vi "Raman Live Tool Set v10.0.0.vi"(1 "Exit":bool, 2 "LiveData":dbl[][](array[numeric]), 3 "RemoteIndicator":bool) -> ()   [LabVIEW 2010]
uses:
  subvi/_TypeDefs/MapFunctions.ctl
  <vilib>/Utility/miscctls.llb/LVPointTypeDef.ctl
  <vilib>/Utility/miscctls.llb/LVStringsAndValuesArrayTypeDef.ctl
  <vilib>/Utility/inputDevices.llb/closeKeyboard.vi
  <vilib>/Utility/inputDevices.llb/keyboardAcquire.vi
  <vilib>/Utility/file.llb/Read From Spreadsheet File (DBL).vi
  <vilib>/Analysis/NI_AALBase.lvlib
panel:
  out "XY Full Interpol.":cluster{dbl, dbl}[](array[cluster])
  out "Axes":T1
  in  "SpectrumNoise":dbl caption="Noise?"
  in  "MapFunction":T2 caption="Mapping function" items=["Total"=0, "Peak"=4, "Area"=2, "Value"=1, "Ratio"=3]
  in  "CreateMap":bool
  in  "SpectrumX":u16(ring) caption="X"
  in  "SpectrumY":u16(ring) caption="Y"
  out "Spectrum":cluster{dbl[], dbl[]}(graph) caption="Current Spectrum"
  in  "MapKeyboard":bool
  in  "MapEditColor":bool caption="Edit Color"
  in  "MapFlipColor":bool caption="Flip Color"
  in  "MapInterpolate":bool
  in  "MapSaveData":bool
  out "Map":dbl[][](graph)
  out "LoadingSpectra":bool
  in  "SourceFile":path caption="Mapping File"
  in  "MapCursorDummy":bool
  out "XY Unique":cluster{"X Unique":dbl[], "Y Unique":dbl[]}
  out "XY Full":cluster{dbl, dbl}[](array[cluster])
  out "Intensities (2D)":dbl[][](array[numeric])
  out "Wavelengths (1D)":dbl[](array[numeric])
  in  "MapColorSlider":cluster{i32, i32, i32, i32, i32, i32, i32}(slide) scale=-6.0..134.0
  out "MapColorTable":u32[](array[numeric])=[0, 196608, 393216, 589824, 786432, 983040, 1179648, 1376256, 1572864, 1769472, 1966080, 2162688, 2359296, 2555904, 2752512, 2949120, 3145728, 3342336, 3538944, 3735552, 3932160, 4128768, 4325376, 4521984, 4718592, 4915200, 5111808, 5308416, 5505024, 5701632, 5898240, 6094848, 6291456, 6488064, 6684672, 6881280, 7077888, 7274496, 7471104, 7667712, 7864320, 8060928, 8257536, 8454144, 8650752, 8847360, 9043968, 9240576, 9437184, 9633792, 9830400, 10027008, 10223616, 10420224, 10616832, 10813440, 11010048, 11206656, 11403264, 11599872, 11796480, 11993088, 12189696, 12386304, 12582912, 12779520, 12976128, 13172736, 13369344, 13565952, 13762560, 13959168, 14155776, 14352384, 14548992, 14745600, 14942208, 15138816, 15335424, 15532032, 15728640, 15925248, 16121856, 16318464, 16515072, 16711680, 16712448, 16713216, 16713984, 16714752, 16715520, 16716288, 16717056, 16717824, 16718592, 16719360, 16720128, 16720896, 16721664, 16722432, 16723200, 16723968, 16724736, 16725504, 16726272, 16727040, 16727808, 16728576, 16729344, 16730112, 16730880, 16731648, 16732416, 16733184, 16733952, 16734720, 16735488, 16736256, 16737024, 16737792, 16738560, 16739328, 16740096, 16740864, 16741632, 16742400, 16743168, 16743936, 16744704, 16745472, 16746240, 16747008, 16747776, 16748544, 16749312, 16750080, 16750848, 16751616, 16752384, 16753152, 16753920, 16754688, 16755456, 16756224, 16756992, 16757760, 16758528, 16759296, 16760064, 16760832, 16761600, 16762368, 16763136, 16763904, 16764672, 16765440, 16766208, 16766976, 16767744, 16768512, 16769280, 16770048, 16770816, 16771584, 16772352, 16773120, 16773888, 16774656, 16775424, 16776192, 16776960, 16776963, 16776966, 16776969, 16776972, 16776975, 16776977, 16776980, 16776983, 16776986, 16776989, 16776992, 16776995, 16776998, 16777001, 16777004, 16777007, 16777009, 16777012, 16777015, 16777018, 16777021, 16777024, 16777027, 16777030, 16777033, 16777036, 16777038, 16777041, 16777044, 16777047, 16777050, 16777053, 16777056, 16777059, 16777062, 16777065, 16777068, 16777070, 16777073, 16777076, 16777079, 16777082, 16777085, 16777088, 16777091, 16777094, 16777097, 16777100, 16777102, 16777105, 16777108, 16777111, 16777114, 16777117, 16777120, 16777123, 16777126, 16777129, 16777132, 16777134, 16777137, 16777140, 16777143, 16777146, 16777149, 16777152, 16777155, 16777158, 16777161, 16777163, 16777166, 16777169, 16777172, 16777175, 16777178, 16777181, 16777184, 16777187, 16777190, 16777193, 16777195, 16777198, 16777201, 16777204, 16777207]
  out "MapZBounds":cluster{dbl, dbl}
  out "MapData (2D)":dbl[][](array[numeric])
  # "Cursor"
  # "Spectrum"
  # "Raman Live Tool Set"
  # "by A. Schmitz-Wunderlich, P. Candeloro"
  # "Cursor"
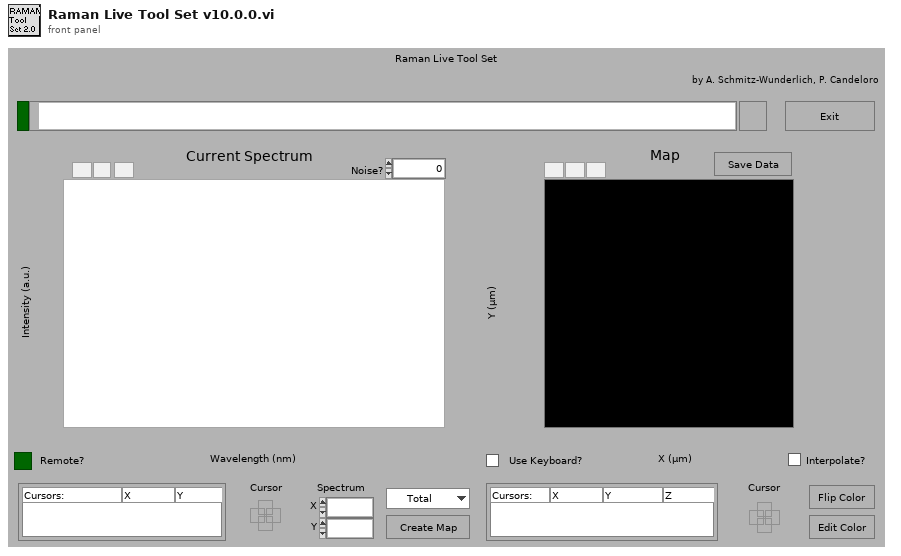
[diagram p1: front panel]
types:
  T1 = cluster{"X":cluster{"Offset":dbl, "Step Size":dbl, "Step Count":i32}, "Y":cluster{"Offset":dbl, "Step Size":dbl, "Step Count":i32}}
  T2 = typedef "MapFunctions.ctl" = u16
  T3 = typedef "LVPointTypeDef.ctl" = cluster{"Horizontal":i16, "Vertical":i16}
  T4 = enum8{"Enabled", "Disabled", "Disabled and Grayed Out"}
  T5 = enum16{"0", "1", "2", "3", "4", "5", "6", "7", "8", "9", "A", "B", "C", "D", "E", "F", "G", "H", "I", "J", "K", "L", "M", "N", "O", "P", "Q", "R", "S", "T", "U", "V", "W", "X", "Y", "Z", "F1", "F2", "F3", "F4", "F5", "F6", "F7", "F8", "F9", "F10", "F11", "F12", "F13", "F14", "F15", "ADD", "BACK", "BACKSLASH", "CAPITAL", "COMMA", "DECIMAL", "DELETE", "DIVIDE", "DOWN", "END", "EQUALS", "ESCAPE", "GRAVE (`)", "HOME", "INSERT", "LBRACKET", "LCONTROL", "LEFT", "L ALT", "LSHIFT", "LWIN", "MINUS", "MULTIPLY", "NEXT", "NUMLOCK", "NUMPAD_0", "NUMPAD_1", "NUMPAD_2", "NUMPAD_3", "NUMPAD_4", "NUMPAD_5", "NUMPAD_6", "NUMPAD_7", "NUMPAD_8", "NUMPAD_9", "PAUSE", "PERIOD", "PRIOR (PG UP)", "RBRACKET", "RCONTROL", "RETURN", "RIGHT", "R ALT", "RSHIFT", "RWIN", "SCROLL", "SEMICOLON", "SLASH", "SPACE", "SUBTRACT", "TAB", "UP", "ENTER (num pad)", "' (quote)"}
  T6 = enum16{"0", "1", "2", "3", "4", "5", "6", "7", "8", "9", "A", "B", "C", "D", "E", "F", "G", "H", "I", "J", "K", "L", "M", "N", "O", "P", "Q", "R", "S", "T", "U", "V", "W", "X", "Y", "Z", "F1", "F2", "F3", "F4", "F5", "F6", "F7", "F8", "F9", "F10", "F11", "F12", "F13", "F14", "F15", "ADD", "BACK", "BACKSLASH", "CAPITAL", "COMMA", "DECIMAL", "DELETE", "DIVIDE", "DOWN", "END", "EQUALS", "ESCAPE", "GRAVE (`)", "HOME", "INSERT", "LBRACKET", "LCONTROL", "LEFT", "L ALT", "LSHIFT", "LWIN", "MINUS", "MULTIPLY", "NEXT", "NUMLOCK", "NUMPAD_0", "NUMPAD_1", "NUMPAD_2", "NUMPAD_3", "NUMPAD_4", "NUMPAD_5", "NUMPAD_6", "NUMPAD_7", "NUMPAD_8", "NUMPAD_9", "PAUSE", "PERIOD", "PRIOR (PG UP)", "RBRACKET", "RCONTROL", "RETURN", "RIGHT", "R ALT", "RSHIFT", "RWIN", "SCROLL", "SEMICOLON", "SLASH", "SPACE", "SUBTRACT", "TAB", "UP", "ENTER (num pad)", "' (quote)"}[]
  T7 = cluster{"Name":string, "Color":u32, "Style":u8, "Point Style":u8, "Name Visible":bool, "Allow Drag":bool, "Cursor Mode":u32, "Plot":i32, "Index":i32, "Position":cluster{"X":dbl, "Y":dbl}, "X Scale":u32, "Y Scale":u32, "Watch Plots":i32[], "Watch All Plots":bool, "Plot Area":i32, "Label Offset":cluster{"X":dbl, "Y":dbl}}
  T8 = cluster{"Name":string, "Color":u32, "Style":u8, "Point Style":u8, "Name Visible":bool, "Allow Drag":bool, "Cursor Mode":u32, "Plot":i32, "Index":i32, "Position":cluster{"X":dbl, "Y":dbl}, "X Scale":u32, "Y Scale":u32, "Watch Plots":i32[], "Watch All Plots":bool, "Plot Area":i32, "Label Offset":cluster{"X":dbl, "Y":dbl}}[]
  T9 = typedef "LVCursorListTypeDef.ctl" = cluster{"Name":string, "Color":u32, "Style":u8, "Point Style":u8, "Name Visible":bool, "Allow Drag":bool, "Cursor Mode":u32, "Plot":i32, "Index":i32, "Position":cluster{"X":dbl, "Y":dbl}, "X Scale":u32, "Y Scale":u32, "Watch Plots":i32[], "Watch All Plots":bool, "Plot Area":i32, "Label Offset":cluster{"X":dbl, "Y":dbl}}[]
  T10 = typedef "LVPointDoubleTypeDef.ctl" = cluster{"Cursor X":dbl, "Cursor Y":dbl}
  T11 = typedef "LVStringsAndValuesArrayTypeDef.ctl" = cluster{"String":string, "Value":ext}[]
  T12 = enum32{"invalid app kind", "Development System", "Run Time System", "Student Edition", "Embedded LabVIEW", "Evaluation", "Custom"}
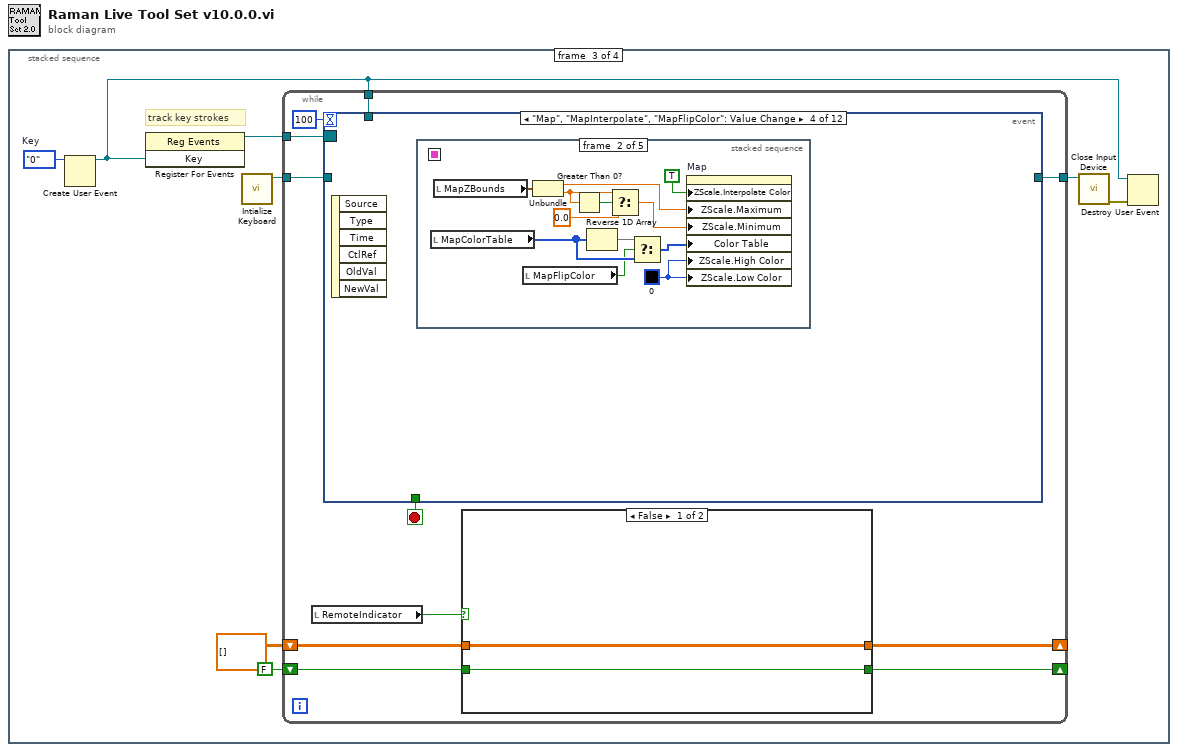
[diagram p0: block diagram]
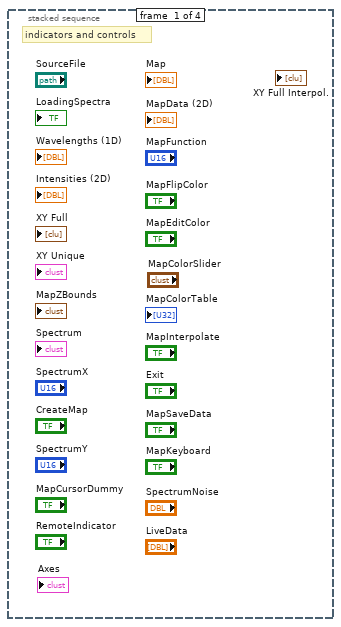
[diagram p2: hidden frame]
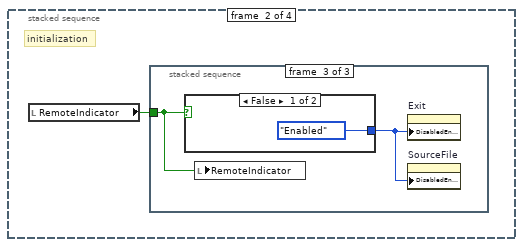
[diagram p3: hidden frame]
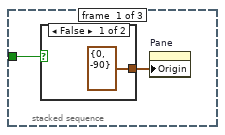
[diagram p4: hidden frame]
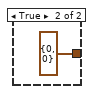
[diagram p5: hidden frame]
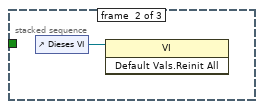
[diagram p6: hidden frame]
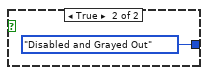
[diagram p7: hidden frame]
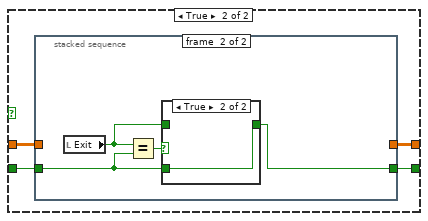
[diagram p8: hidden frame]
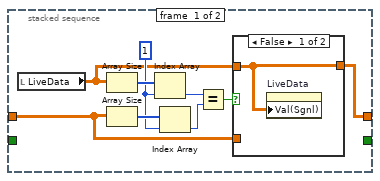
[diagram p9: hidden frame]
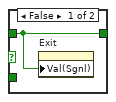
[diagram p11: hidden frame]
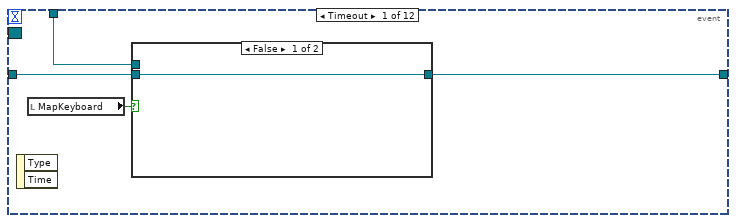
[diagram p12: hidden frame]
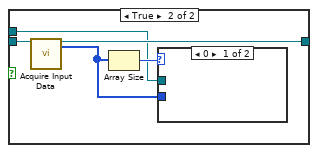
[diagram p13: hidden frame]
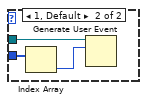
[diagram p14: hidden frame]
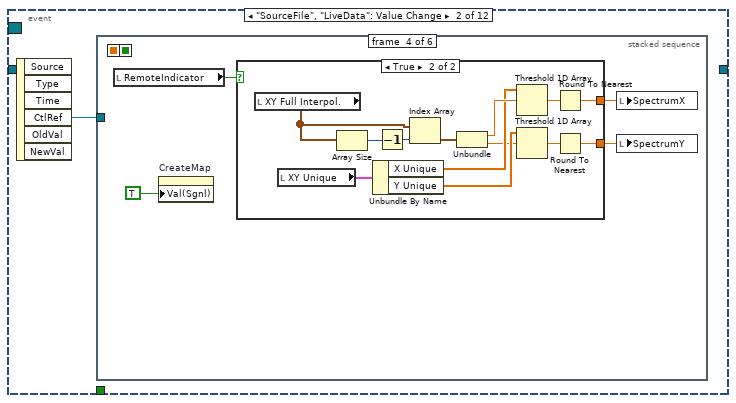
[diagram p15: hidden frame]
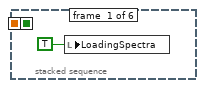
[diagram p16: hidden frame]
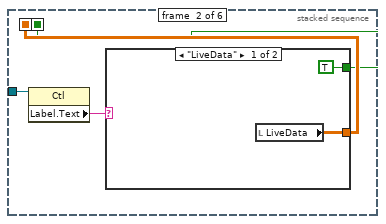
[diagram p17: hidden frame]
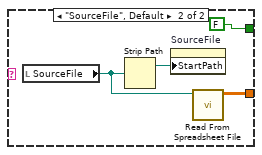
[diagram p18: hidden frame]
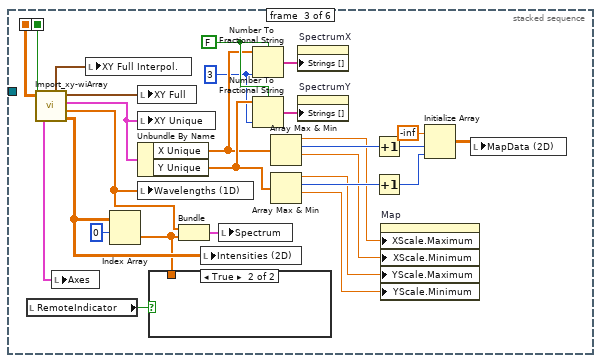
[diagram p19: hidden frame]
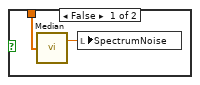
[diagram p20: hidden frame]
diagram:
  n1 = stacked-sequence {
    frame #0 {
      # "indicators and controls"
    }
    frame #1 {
      # "initialization"
      n2 = local read "RemoteIndicator"() -> (w1:bool)
      n3 = stacked-sequence {
        tunnel: w1 -> [w2 _ w7]
        frame #0 {
          n4 = case shown="False" w2 {
            tunnel: [T3 {"Horizontal"=0, "Vertical"=-90} ("Origin") T3 {"Horizontal"=0, "Vertical"=0} ("Origin")] -> w3
            frame False {
            }
            frame True {
            }
          }
          n5 = property on="Pane" class="Pane"("Origin"=w3) -> ()  [unwired: 2 in, 2 out]
        }
        frame #1 {
          n6 = control-ref of="Dieses VI"() -> (w6:refnum<vi>)
          n7 = invoke class="VI" method="Default Vals.Reinit All"(reference=w6) -> ()  [unwired: 2 in, 3 out]
        }
        frame #2 {
          n8 = case shown="False" w7 {
            tunnel: [T4."Enabled" ("Deaktiviert") T4."Disabled and Grayed Out" ("Deaktiviert")] -> w8
            frame False {
            }
            frame True {
            }
          }
          n9 = local write "RemoteIndicator"(w7) -> ()
          n10 = property on="Exit" class="Bool (strict)"("DisabledEnum"=w8) -> ()  [unwired: 2 in, 2 out]
          n11 = property on="SourceFile" class="Path"("DisabledEnum"=w8) -> ()  [unwired: 2 in, 2 out]
        }
      }
    }
    frame #2 {
      w18 = T5."0"  # Key
      # "track key strokes"
      n12 = Create User Event(user event datatype=w18) -> (user event=w15:refnum<user-event>)  [unwired: 1 in, 1 out]
      n13 = register-events(w15) -> (reference out=w16:refnum<event-registration>)  [unwired: 2 in, 1 out]
      n14 = call <vilib>:"Intialize Keyboard.vi"() -> ("device ID"=w14:refnum<k1>)  [unwired: 10 in, 1 out]
      n15 = while {
        tunnel: w16 -> [w28]
        tunnel: w15 -> [w27]
        tunnel: w14 -> [w26]
        tunnel: [w25] -> w13
        shift-right: [w21] -> _
        shift-left: dbl[][] [] ("LiveData") -> [w22]
        shift-right: [w19] -> _
        shift-left: FALSE -> [w20]
        stop <- w29 stop-if-true
        n16 = local read "RemoteIndicator"() -> (w23:bool)
        n17 = event shown="[3] \"Map\", \"MapInterpolate\", \"MapFlipColor\": Value Change" {
          selector: w28 -> [_ _ _ _ _ _ _ _ _ _ _ _]
          dyn-events: _ -> [_ _ _ _ _ _ _ _ _ _ _ _]
          timeout: 100 -> [_ _ _ _ _ _ _ _ _ _ _ _]
          tunnel: [_ _ _ _ _ _ _ _ _ _ _ w313] -> w29
          tunnel: w27 -> [w56 _ _ _ _ _ _ _ _ _ _ _]
          tunnel: w26 -> [w55 _ _ _ _ _ _ _ _ _ _ _]
          tunnel: [w53 _ _ _ _ _ _ _ _ _ _ _] -> w25
          event Timeout {
            n18 = event-data() -> ()  [unwired: 1 in, 2 out]
            n19 = local read "MapKeyboard"() -> (w54:bool)
            n20 = case shown="False" w54 {
              tunnel: [w57 w62] -> w53
              tunnel: w56 -> [_ w59]
              tunnel: w55 -> [w57 w58]
              frame False {
              }
              frame True {
                n21 = call-poly <vilib>:"Acquire Input Data.vi"("device ID"=w58) -> ("device ID"=w62:refnum<k1>, "keys pressed"=w61:T6)  [unwired: 16 in, 1 out]
                n22 = Array Size(array=w61) -> (size(s)=w60:i32)
                n23 = case shown="0" w60 {
                  tunnel: w59 -> [_ w65]
                  tunnel: w61 -> [_ w63]
                  frame 0 {
                  }
                  frame 1, Default {
                    n24 = Index Array(array=w63) -> (element=w64:T5)  [unwired: 1 in]
                    n25 = Generate User Event(user event=w65, event data cluster=w64) -> ()  [unwired: 1 in, 2 out]
                  }
                }
              }
            }
          }
          event "SourceFile", "LiveData": Value Change {
            n26 = event-data() -> ("CtlRef"=w66:refnum<vi>)  [unwired: 1 in, 5 out]
            n27 = stacked-sequence {
              seq-local: [_ w69 _ _ _ _] -> [_ _ w87 _ _ _]
              seq-local: [_ w68 _ _ _ _] -> [_ _ w80 _ _ _]
              tunnel: w66 -> [_ w71 _ _ _ _]
              frame #0 {
                n28 = local write "LoadingSpectra"(TRUE ("Loading\nSpectra")) -> ()
              }
              frame #1 {
                n29 = property class="Ctl"(reference=w71) -> ("Label.Text"=w70:string)  [unwired: 1 in, 2 out]
                n30 = case shown="\"LiveData\"" w70 {
                  tunnel: [w73 w75] -> w69
                  tunnel: [TRUE FALSE] -> w68
                  frame "LiveData" {
                    n31 = local read "LiveData"() -> (w73:dbl[][])
                  }
                  frame "SourceFile", Default {
                    n32 = local read "SourceFile"() -> (w76:path)
                    n33 = Strip Path(path=w76) -> (stripped path=w77:path)  [unwired: 1 out]
                    n34 = property on="SourceFile" class="Path"("StartPath"=w77) -> ()  [unwired: 2 in, 2 out]
                    n35 = call-poly <vilib>:"Read From Spreadsheet File.vi"("file path (dialog if empty)"=w76) -> ("all rows"=w75:dbl[][])  [unwired: 6 in, 4 out]
                  }
                }
              }
              frame #2 {
                w94 = i16 3 ("Genauigkeit (6)")
                w101 = FALSE ("Systemdezimalzeichen verwenden (T)")
                n36 = local read "RemoteIndicator"() -> (w81:bool)
                n37 = call "Import_xy-wiArray.vi"("InputArray"=w87, "Uniform"=w80) -> ("XY Full"=w79:cluster{dbl, dbl}[], "XY Unique"=w84:cluster{"X Unique":dbl[], "Y Unique":dbl[]}, "Wavelength"=w85:dbl[], "Intensity"=w86:dbl[][], "XY Full Interpol."=w78:cluster{dbl, dbl}[], "Axes"=w82:T1)
                n38 = local write "Axes"(w82) -> ()
                n39 = local write "XY Full Interpol."(w78) -> ()
                n40 = Index Array(array=w86, index (row)=0 ("Index (Zeile)")) -> (element=w83:dbl[])  [unwired: 1 in]
                n41 = local write "XY Full"(w79) -> ()
                n42 = local write "XY Unique"(w84) -> ()
                n43 = Unbundle By Name(w84) -> ("X Unique"=w95:dbl[], "Y Unique"=w96:dbl[])
                n44 = local write "Wavelengths (1D)"(w85) -> ()
                n45 = case shown="True" w81 {
                  tunnel: w83 -> [w106 _]
                  frame False {
                    n46 = call <vilib>:"Median.vi"("X"=w106) -> ("median"=w107:dbl)  [unwired: 1 out]
                    n47 = local write "SpectrumNoise"(w107) -> ()
                  }
                  frame True {
                  }
                }
                n48 = Bundle("Wavelength"=w85, "Intensity"=w83) -> (w105:cluster{"Wavelength":dbl[], "Intensity":dbl[]})  [unwired: 1 in]
                n49 = local write "Intensities (2D)"(w86) -> ()
                n50 = local write "Spectrum"(w105) -> ()
                n51 = Number To Fractional String(use system decimal point (T)=w101, number=w95, precision (6)=w94) -> (F-format string=w98:string[])  [unwired: 1 in]
                n52 = Number To Fractional String(use system decimal point (T)=w101, number=w96, precision (6)=w94) -> (F-format string=w97:string[])  [unwired: 1 in]
                n53 = Array Max & Min(array=w95) -> (max value=w91:dbl, max index (indices)=w93:i32, min value=w90:dbl)  [unwired: 1 out]
                n54 = Array Max & Min(array=w96) -> (max value=w89:dbl, max index (indices)=w92:i32, min value=w88:dbl)  [unwired: 1 out]
                n55 = property on="SpectrumX" class="Ring (strict)"("Strings []"=w98) -> ()  [unwired: 2 in, 2 out]
                n56 = property on="SpectrumY" class="Ring (strict)"("Strings []"=w97) -> ()  [unwired: 2 in, 2 out]
                n57 = Increment(x=w93) -> (x+1=w102:i32)
                n58 = Increment(x=w92) -> (x+1=w103:i32)
                n59 = property on="Map" class="IntGraph (strict)"("XScale.Maximum"=w91, "XScale.Minimum"=w90, "YScale.Maximum"=w89, "YScale.Minimum"=w88) -> ()  [unwired: 2 in, 2 out]
                n60 = Initialize Array(-inf, w102, w103) -> (w100:dbl[][])
                n61 = local write "MapData (2D)"(w100) -> ()
              }
              frame #3 {
                n62 = local read "RemoteIndicator"() -> (w111:bool)
                n63 = property on="CreateMap" class="Bool (strict)"("Val(Sgnl)"=TRUE ("Wert (signalisierend)")) -> ()  [unwired: 2 in, 2 out]
                n64 = case shown="True" w111 {
                  tunnel: [w112 w113] -> w110
                  tunnel: [w112 w114] -> w109
                  frame False {
                    w112 = 0
                  }
                  frame True {
                    n65 = local read "XY Full Interpol."() -> (w122:cluster{dbl, dbl}[])
                    n66 = local read "XY Unique"() -> (w125:cluster{"X Unique":dbl[], "Y Unique":dbl[]})
                    n67 = Array Size(array=w122) -> (size(s)=w124:i32)
                    n68 = Unbundle By Name(w125) -> ("X Unique"=w118:dbl[], "Y Unique"=w117:dbl[])
                    n69 = Decrement(x=w124) -> (x-1=w123:i32)
                    n70 = Index Array(array=w122, index=w123) -> (element=w121:cluster{dbl, dbl})
                    n71 = Unbundle(w121) -> (w119:dbl, w116:dbl)
                    n72 = Threshold 1D Array(2:w119, 3:w118) -> (0:w120:dbl)  [unwired: 1 in]
                    n73 = Threshold 1D Array(2:w116, 3:w117) -> (0:w115:dbl)  [unwired: 1 in]
                    n74 = Round To Nearest(number=w120) -> (nearest integer value=w113:dbl)
                    n75 = Round To Nearest(number=w115) -> (nearest integer value=w114:dbl)
                  }
                }
                n76 = local write "SpectrumX"(w110) -> ()
                n77 = local write "SpectrumY"(w109) -> ()
              }
              frame #4 {
                w135 = i8 2 ("y")
                w143 = T7 {"Name"="cursor", "Color"=1985280, "Style"=2, "Point Style"=6, "Name Visible"=FALSE, "Allow Drag"=TRUE, "Cursor Mode"=0, "Plot"=0, "Index"=0, "Position"={"X"=0.0, "Y"=0.0}, "X Scale"=0, "Y Scale"=0, "Watch Plots"=[], "Watch All Plots"=FALSE, "Plot Area"=0, "Label Offset"={"X"=0.0, "Y"=0.0}}  # cursorConst
                n78 = local read "Axes"() -> (w139:T1)
                n79 = Unbundle By Name(w139) -> ("X.Offset"=w138:dbl, "X.Step Size"=w137:dbl, "Y.Offset"=w134:dbl, "Y.Step Size"=w136:dbl)
                n80 = Divide(x=w137, y=w135) -> (x/y=w133:dbl)
                n81 = Divide(x=w136, y=w135) -> (x/y=w132:dbl)
                n82 = Add(x=w138, y=w133) -> (x+y=w130:dbl)
                n83 = Add(x=w134, y=w132) -> (x+y=w131:dbl)
                n84 = Bundle(w130, w131) -> (w128:cluster{dbl, dbl})  [unwired: 1 in]
                n85 = Bundle By Name(cluster=w143, "Name"="Spot", "Cursor Mode"=u32 0, "Position"=w128) -> (w127:T7)
                n86 = Build Array(w127) -> (w126:T8)
                n87 = property on="Map" class="IntGraph (strict)"("CrsrLis"=w126, "Cursor.Cursor Style"=u8 8, "Cursor.Cursor Point Style"=u8 5, "Cursor.Cursor Color"=u32 16448250 ("Color")) -> ()  [unwired: 2 in, 2 out]
              }
              frame #5 {
                n88 = local write "LoadingSpectra"(FALSE ("Loading\nSpectra")) -> ()
              }
            }
          }
          event "CreateMap": Value Change {
            n89 = event-data() -> ("NewVal"=w146:bool)  [unwired: 1 in, 5 out]
            n90 = case shown="True" w146 {
              frame False {
              }
              frame True {
                n91 = stacked-sequence {
                  frame #0 {
                    n92 = property on="Spectrum" class="XYGraph (strict)"() -> ("CrsrList"=w155:T9)  [unwired: 2 in, 2 out]
                    n93 = local read "XY Full Interpol."() -> (w148:cluster{dbl, dbl}[])
                    n94 = local read "SpectrumNoise"() -> (w151:dbl)
                    n95 = local read "Intensities (2D)"() -> (w150:dbl[][])
                    n96 = local read "Wavelengths (1D)"() -> (w162:dbl[])
                    n97 = local read "MapFunction"() -> (w152:T2)
                    n98 = Index Array(array=w155, index=0 ("Index")) -> (element=w158:T7)
                    n99 = Index Array(array=w155, index=1 ("Index")) -> (element=w159:T7)
                    n100 = Unbundle By Name(w158) -> ("Position.X"=w154:dbl)
                    n101 = Unbundle By Name(w159) -> ("Position.X"=w153:dbl)
                    n102 = local read "XY Unique"() -> (w147:cluster{"X Unique":dbl[], "Y Unique":dbl[]})
                    n103 = Subtract(x=w150, y=w151) -> (x-y=w149:dbl[][])
                    n104 = call "Map_spectra2MapData.vi"("Intensity"=w149, "Wavelength"=w162, "XY Unique"=w147, "XY Full"=w148, "MapFunction"=w152, "X1"=w154, "X2"=w153) -> ("MapZBounds"=w160:cluster{sgl, sgl}, "MapData"=w161:sgl[][])  [unwired: 2 in]
                    n105 = local write "MapZBounds"(w160) -> ()
                    n106 = local write "MapData (2D)"(w161) -> ()
                    n107 = property on="Map" class="IntGraph (strict)"("Val(Sgnl)"=w161) -> ()  [unwired: 2 in, 2 out]
                  }
                  frame #1 {
                    n108 = local read "SpectrumX"() -> (w164:u16)
                    n109 = local write "CreateMap"(FALSE ("Value")) -> ()
                    n110 = property on="SpectrumX" class="Ring (strict)"("Val(Sgnl)"=w164) -> ()  [unwired: 2 in, 2 out]
                  }
                }
              }
            }
          }
          event "Map", "MapInterpolate", "MapFlipColor": Value Change {
            n111 = event-data() -> ()  [unwired: 1 in, 6 out]
            n112 = stacked-sequence {
              seq-local: [w165 _ _ _ _] -> [_ _ w190 _ _]
              frame #0 {
                n113 = local read "MapInterpolate"() -> (w170:bool)
                n114 = local read "MapData (2D)"() -> (w169:dbl[][])
                n115 = local read "XY Unique"() -> (w166:cluster{"X Unique":dbl[], "Y Unique":dbl[]})
                n116 = local read "Axes"() -> (w168:T1)
                n117 = case shown="True" w170 {
                  tunnel: [w172 w176] -> w167
                  tunnel: w169 -> [w172 w177]
                  tunnel: w168 -> [w171 _]
                  tunnel: w166 -> [_ w174]
                  tunnel: [w171 w173] -> w165
                  frame False {
                  }
                  frame True {
                    n118 = call "Map_interpolateXYZ.vi"("Level"=3, "MapData (2D)"=w177, "XY Unique"=w174) -> ("Z Interpoliert"=w176:dbl[][], "Axes"=w173:T1)  [unwired: 1 out]
                  }
                }
                n119 = local write "Map"(w167) -> ()
              }
              frame #1 {
                w185 = u32 0 ("Color")
                n120 = local read "MapColorTable"() -> (w183:u32[])
                n121 = local read "MapZBounds"() -> (w184:cluster{dbl, dbl})
                n122 = local read "MapFlipColor"() -> (w182:bool)
                n123 = Unbundle(w184) -> (w188:dbl, w181:dbl)
                n124 = Greater Than 0?(x=w181) -> (x > 0?=w179:bool)
                n125 = Reverse 1D Array(array=w183) -> (reversed array=w187:u32[])
                n126 = Select(t=w181, s=w179, f=0.0) -> (s? t:f=w178:dbl)
                n127 = Select(t=w187, s=w182, f=w183) -> (s? t:f=w186:u32[])
                n128 = property on="Map" class="IntGraph (strict)"("ZScale.Interpolate Color"=TRUE ("Z Scale.Interpolate Color"), "ZScale.Maximum"=w188, "ZScale.Minimum"=w178, "Color Table"=w186, "ZScale.High Color"=w185, "ZScale.Low Color"=w185) -> ()  [unwired: 2 in, 2 out]
              }
              frame #2 {
                n129 = Unbundle By Name(w190) -> ("X.Offset"=w194:dbl, "X.Step Size"=w193:dbl, "Y.Offset"=w192:dbl, "Y.Step Size"=w191:dbl)
                n130 = property on="Map" class="IntGraph (strict)"("XScale.Offset"=w194, "XScale.Multiplier"=w193, "YScale.Offset"=w192, "YScale.Multiplier"=w191) -> ()  [unwired: 2 in, 2 out]
              }
              frame #3 {
                w195 = u8 1 ("X-Achse.Achsenanpassung")
                n131 = property on="Map" class="IntGraph (strict)"("XScale.ScaleFit"=w195, "YScale.ScaleFit"=w195, "ZScale.ScaleFit"=u8 0 ("Z-Achse.Achsenanpassung")) -> ()  [unwired: 2 in, 2 out]
              }
              frame #4 {
                n132 = local read "SpectrumX"() -> (w197:u16)
                n133 = property on="SpectrumX" class="Ring (strict)"("Val(Sgnl)"=w197) -> ()  [unwired: 2 in, 2 out]
              }
            }
          }
          event "MapEditColor": Value Change {
            n134 = event-data() -> ("NewVal"=w198:bool)  [unwired: 1 in, 5 out]
            n135 = case shown="True" w198 {
              frame False {
              }
              frame True {
                n136 = flat-sequence {
                  frame #0 {
                    n137 = local read "MapColorTable"() -> (w199:u32[])
                    n138 = call "MapColor_makeRamp.vi"("ColorMap\narray IN"=w199) -> ("ColorMap\narray OUT"=w200:u32[])
                    n139 = local write "MapColorTable"(w200) -> ()
                  }
                  frame #1 {
                    n140 = local read "MapData (2D)"() -> (w202:dbl[][])
                    n141 = local write "MapEditColor"(FALSE ("Value")) -> ()
                    n142 = property on="Map" class="IntGraph (strict)"("Val(Sgnl)"=w202) -> ()  [unwired: 2 in, 2 out]
                  }
                }
              }
            }
          }
          event "MapSaveData": Value Change {
            n143 = event-data() -> ("NewVal"=w203:bool)  [unwired: 1 in, 5 out]
            n144 = case shown="True" w203 {
              frame False {
              }
              frame True {
                n145 = flat-sequence {
                  frame #0 {
                    n146 = property on="MapFunction" class="Ring (strict)"() -> ("RingText.Text"=w205:string)  [unwired: 2 in, 2 out]
                    n147 = local read "SourceFile"() -> (w204:path)
                    n148 = control-ref of="Spectrum"() -> (w206:refnum<vi>)
                    n149 = call "Export_mapFileName.vi"("MapFunctionStr"=w205, "Spectrum"=w206, "SourceFile"=w204) -> ("Dateipfad"=w207:path)
                    n150 = local read "XY Full"() -> (w208:cluster{dbl, dbl}[])
                    n151 = local read "Map"() -> (w209:dbl[][])
                    n152 = call "Export_map2Text.vi"("MapData (2D)"=w209, "XY Full"=w208, "ExportPath"=w207) -> ()  [unwired: 1 in]
                  }
                  frame #1 {
                    n153 = local write "MapSaveData"(FALSE ("Value")) -> ()
                    n154 = Wait (ms)(milliseconds to wait=u32 300) -> ()  [unwired: 1 out]
                  }
                }
              }
            }
          }
          event Value Change {
            n155 = event-data() -> ()  [unwired: 1 in, 6 out]
            n156 = local read "MapFunction"() -> (w212:T2)
            n157 = control-ref of="Spectrum"() -> (w213:refnum<vi>)
            n158 = call "SpectrumCursor_init.vi"("MapFunction"=w212, "Spectrum"=w213) -> ()  [unwired: 1 in]
          }
          event "SpectrumY", "SpectrumX", "SpectrumNoise": Value Change {
            n159 = event-data() -> ()  [unwired: 1 in, 6 out]
            n160 = local read "XY Unique"() -> (w228:cluster{"X Unique":dbl[], "Y Unique":dbl[]})
            n161 = local read "SpectrumX"() -> (w221:u16)
            n162 = local read "SpectrumY"() -> (w222:u16)
            n163 = Unbundle By Name(w228) -> ("X Unique"=w224:dbl[], "Y Unique"=w223:dbl[])
            n164 = local read "XY Full Interpol."() -> (w214:cluster{dbl, dbl}[])
            n165 = Index Array(array=w224, index=w221) -> (element=w233:dbl)
            n166 = Index Array(array=w223, index=w222) -> (element=w232:dbl)
            n167 = Bundle(cluster=cluster{dbl, dbl} {0.0, 0.0} ("Element"), w233, w232) -> (w217:cluster{dbl, dbl})
            n168 = property on="Map" class="IntGraph (strict)"("Cursor.Cursor Position"=w217) -> ()  [unwired: 2 in, 2 out]
            n169 = while {
              tunnel: w214 -> [w240] mode=indexing
              tunnel: w217 -> [w241]
              tunnel: [w239] -> w219
              tunnel: [w236] -> w216
              tunnel: w214 -> [w237]
              i -> [w239]
              stop <- w234 stop-if-true
              n170 = Array Size(array=w237) -> (size(s)=w238:i32)
              n171 = Equal?(x=w240, y=w241) -> (x = y?=w236:bool)
              n172 = Greater?(x=w239, y=w238) -> (0:w235:bool)
              n173 = Or(x=w235, y=w236) -> (x .or. y?=w234:bool)
            }
            n174 = local read "SpectrumNoise"() -> (w227:dbl)
            n175 = local read "Intensities (2D)"() -> (w230:dbl[][])
            n176 = local read "Wavelengths (1D)"() -> (w231:dbl[])
            n177 = Select(t=w219, s=w216, f=u8 0) -> (s? t:f=w215:i32)
            n178 = Index Array(array=w230, index (row)=w215) -> (element=w226:dbl[])  [unwired: 1 in]
            n179 = Subtract(x=w226, y=w227) -> (x-y=w225:dbl[])
            n180 = Bundle("Wavelengths (1D)"=w231, w225) -> (w229:cluster{"Wavelengths (1D)":dbl[], dbl[]})  [unwired: 1 in]
            n181 = local write "Spectrum"(w229) -> ()
          }
          event "Map": Cursor Release; "MapCursorDummy": Value Change {
            n182 = event-data() -> ()  [unwired: 1 in, 4 out]
            n183 = property on="Map" class="IntGraph (strict)" props=["Cursor", "Cursor Position", "Cursor", "Cursor Position"]() -> ("Cursor.Cursor Position"=w251:T10)  [unwired: 2 in, 3 out]
            n184 = local read "XY Unique"() -> (w256:cluster{"X Unique":dbl[], "Y Unique":dbl[]})
            n185 = Unbundle By Name(w256) -> ("X Unique"=w244:dbl[], "Y Unique"=w245:dbl[])
            n186 = Unbundle By Name(w251) -> ("Cursor X"=w255:dbl, "Cursor Y"=w254:dbl)
            n187 = Threshold 1D Array(2:w255, 3:w244) -> (0:w250:dbl)  [unwired: 1 in]
            n188 = Threshold 1D Array(2:w254, 3:w245) -> (0:w249:dbl)  [unwired: 1 in]
            n189 = Round To Nearest(number=w250) -> (nearest integer value=w252:dbl)
            n190 = Round To Nearest(number=w249) -> (nearest integer value=w253:dbl)
            n191 = To Unsigned Word Integer(number=w252) -> (unsigned 16bit integer=w242:u16)
            n192 = To Unsigned Word Integer(number=w253) -> (unsigned 16bit integer=w243:u16)
            n193 = Not Equal?(x=w242, y=w250) -> (x != y?=w247:bool)
            n194 = Not Equal?(x=w243, y=w249) -> (x != y?=w248:bool)
            n195 = property on="SpectrumX" class="Ring (strict)"("Val(Sgnl)"=w242) -> ()  [unwired: 2 in, 2 out]
            n196 = property on="SpectrumY" class="Ring (strict)"("Val(Sgnl)"=w243) -> ()  [unwired: 2 in, 2 out]
            n197 = Or(x=w247, y=w248) -> (x .or. y?=w246:bool)
            n198 = case shown="True" w246 {
              tunnel: w245 -> [_ w260]
              tunnel: w244 -> [_ w259]
              tunnel: w243 -> [_ w258]
              tunnel: w242 -> [_ w257]
              frame False {
              }
              frame True {
                n199 = Index Array(array=w259, index=w257) -> (element=w262:dbl)
                n200 = Index Array(array=w260, index=w258) -> (element=w263:dbl)
                n201 = Bundle(w262, w263) -> (w261:cluster{dbl, dbl})  [unwired: 1 in]
                n202 = property on="Map" class="IntGraph (strict)"("Cursor.Cursor Position"=w261) -> ()  [unwired: 2 in, 2 out]
              }
            }
          }
          event "Spectrum": Cursor Release {
            n203 = event-data() -> ()  [unwired: 1 in, 9 out]
            n204 = local read "MapFunction"() -> (w264:T2)
            n205 = control-ref of="Spectrum"() -> (w265:refnum<vi>)
            n206 = call "SpectrumCursor_set.vi"("MapFunction"=w264, "Spectrum"=w265) -> ()
          }
          event User Event {
            n207 = event-data() -> ("Key"=w272:T5)  [unwired: 1 in, 4 out]
            n208 = property on="Map" class="IntGraph (strict)"() -> ("Cursor.Cursor Position"=w273:T10)  [unwired: 2 in, 2 out]
            n209 = local read "Axes"() -> (w266:T1)
            n210 = property on="Map" class="IntGraph (strict)"() -> ("XScale.Maximum"=w277:dbl, "YScale.Maximum"=w276:dbl, "XScale.Minimum"=w275:dbl, "YScale.Minimum"=w274:dbl)  [unwired: 2 in, 2 out]
            n211 = Unbundle By Name(w266) -> ("X.Step Size"=w270:dbl, "Y.Step Size"=w269:dbl)
            n212 = Unbundle By Name(w273) -> ("Cursor X"=w278:dbl, "Cursor Y"=w279:dbl)
            n213 = case shown="\"DOWN\"" w272 {
              tunnel: w275 -> [_ w285 _ _ _]
              tunnel: w277 -> [_ _ w292 _ _]
              tunnel: w276 -> [_ _ _ w299 _]
              tunnel: w274 -> [_ _ _ _ w306]
              tunnel: w278 -> [w283 w284 w291 w303 w310]
              tunnel: w279 -> [w282 w289 w296 w298 w305]
              tunnel: [w282 w289 w296 w302 w309] -> w280
              tunnel: [w283 w288 w295 w303 w310] -> w281
              tunnel: w270 -> [_ w287 w294 _ _]
              tunnel: w269 -> [_ _ _ w300 w307]
              frame "0", Default {
              }
              frame "LEFT" {
                n214 = Subtract(x=w284, y=w287) -> (x-y=w286:dbl)
                n215 = Greater Or Equal?(x=w285, y=w286) -> (x >= y?=w290:bool)
                n216 = Select(t=w284, s=w290, f=w286) -> (s? t:f=w288:dbl)
              }
              frame "RIGHT" {
                n217 = Add(x=w291, y=w294) -> (x+y=w293:dbl)
                n218 = Greater Or Equal?(x=w292, y=w293) -> (x >= y?=w297:bool)
                n219 = Select(t=w293, s=w297, f=w291) -> (s? t:f=w295:dbl)
              }
              frame "UP" {
                n220 = Add(x=w298, y=w300) -> (x+y=w301:dbl)
                n221 = Less Or Equal?(x=w299, y=w301) -> (x <= y?=w304:bool)
                n222 = Select(t=w298, s=w304, f=w301) -> (s? t:f=w302:dbl)
              }
              frame "DOWN" {
                n223 = Subtract(x=w305, y=w307) -> (x-y=w308:dbl)
                n224 = Greater Or Equal?(x=w306, y=w308) -> (x >= y?=w311:bool)
                n225 = Select(t=w305, s=w311, f=w308) -> (s? t:f=w309:dbl)
              }
            }
            n226 = Bundle("Cursor X"=w281, "Cursor Y"=w280) -> (w271:cluster{"Cursor X":dbl, "Cursor Y":dbl})  [unwired: 1 in]
            n227 = local read "MapCursorDummy"() -> (w267:bool)
            n228 = property on="Map" class="IntGraph (strict)"("Cursor.Cursor Position"=w271) -> (error out=w268:errorcluster)  [unwired: 2 in, 1 out]
            n229 = property on="MapCursorDummy" class="Bool (strict)"(error in=w268, "Val(Sgnl)"=w267) -> ()  [unwired: 1 in, 2 out]
          }
          event "Exit": Value Change {
            n230 = event-data() -> ("OldVal"=w312:bool, "NewVal"=w313:bool)  [unwired: 1 in, 4 out]
            n231 = local write "Exit"(w312) -> ()
          }
        }
        n232 = case shown="False" w23 {
          tunnel: w22 -> [w31 w35]
          tunnel: [w31 w34] -> w21
          tunnel: w20 -> [w30 w33]
          tunnel: [w30 w32] -> w19
          frame False {
          }
          frame True {
            n233 = stacked-sequence {
              tunnel: w35 -> [w39 _]
              tunnel: [w38 _] -> w34
              tunnel: w33 -> [_ w47]
              tunnel: [_ w49] -> w32
              frame #0 {
                w42 = 1 ("Index")
                n234 = local read "LiveData"() -> (w40:dbl[][])
                n235 = Array Size(array=w40) -> (size(s)=w43:i32[])
                n236 = Array Size(array=w39) -> (size(s)=w44:i32[])
                n237 = Index Array(array=w43, index=w42) -> (element=w37:i32)
                n238 = Index Array(array=w44, index=w42) -> (element=w36:i32)
                n239 = Equal?(x=w37, y=w36) -> (x = y?=w41:bool)
                n240 = case shown="False" w41 {
                  tunnel: [w45 w46] -> w38
                  tunnel: w39 -> [_ w46]
                  tunnel: w40 -> [w45 _]
                  frame False {
                    n241 = property on="LiveData" class="Arr (strict)"("Val(Sgnl)"=w45) -> ()  [unwired: 2 in, 2 out]
                  }
                  frame True {
                  }
                }
              }
              frame #1 {
                n242 = local read "Exit"() -> (w48:bool)
                n243 = Equal?(x=w48, y=w47) -> (x = y?=w50:bool)
                n244 = case shown="True" w50 {
                  tunnel: [w51 w52] -> w49
                  tunnel: w47 -> [_ w52]
                  tunnel: w48 -> [w51 _]
                  frame False {
                    n245 = property on="Exit" class="Bool (strict)"("Val(Sgnl)"=w51) -> ()  [unwired: 2 in, 2 out]
                  }
                  frame True {
                  }
                }
              }
            }
          }
        }
      }
      n246 = call-poly <vilib>:"Close Input Device.vi"("device ID"=w13) -> ("error out"=w17:errorcluster)  [unwired: 9 in]
      n247 = Destroy User Event(user event=w15, error in=w17) -> ()  [unwired: 1 out]
    }
    frame #3 {
      w316 = T4."Enabled" ("Deaktiviert")
      w317 = T11 [] ("Strings und Werte []")
      w318 = T8 [] ("Cursor List")
      # "reset and shutdown"
      n248 = control-ref of="Dieses VI"() -> (w319:refnum<vi>)
      n249 = invoke class="VI" method="Default Vals.Reinit All"(reference=w319) -> (reference out=w314:refnum<vi>)  [unwired: 2 in, 2 out]
      n250 = property on="SpectrumY" class="Ring (strict)"("StringsAndValues[]"=w317) -> ()  [unwired: 2 in, 2 out]
      n251 = property on="SpectrumX" class="Ring (strict)"("StringsAndValues[]"=w317) -> ()  [unwired: 2 in, 2 out]
      n252 = property on="SourceFile" class="Path"("DisabledEnum"=w316) -> ()  [unwired: 2 in, 2 out]
      n253 = property on="Exit" class="Bool (strict)"("DisabledEnum"=w316) -> ()  [unwired: 2 in, 2 out]
      n254 = property on="Map" class="IntGraph (strict)"("CrsrLis"=w318) -> ()  [unwired: 2 in, 2 out]
      n255 = property on="Spectrum" class="XYGraph (strict)"("CrsrList"=w318) -> ()  [unwired: 2 in, 2 out]
      n256 = property class="App"() -> ("App.Kind"=w315:T12)  [unwired: 2 in, 2 out]
      n257 = case shown="\"Development System\"" w315 {
        tunnel: w314 -> [w320 _]
        frame "invalid app kind", Default {
          n258 = invoke on="Invoke Node" class="VI" method="FP.Close"(reference=w320) -> ()  [unwired: 2 in, 3 out]
        }
        frame "Development System" {
        }
      }
    }
  }
